vi "Read Measurements.vi"(8 "error in (no error)":errorcluster, 11 "PacificPowerSource in":refnum<class "PacificPowerSource.lvclass">) -> (0 "error out":errorcluster, 2 "BaseMeasurements":T1, 3 "PacificPowerSource out":refnum<class "PacificPowerSource.lvclass">)   [LabVIEW 2018, in "AcPwrPlugins.lvlib" / "PacificPowerSource.lvclass"]
uses:
  PacificPowerSource.lvclass
  TypeDefs/Measurements.ctl
  TypeDefs/MeasurementType.ctl
  PacificPowerSource.lvclass/PacificPowerSource.ctl
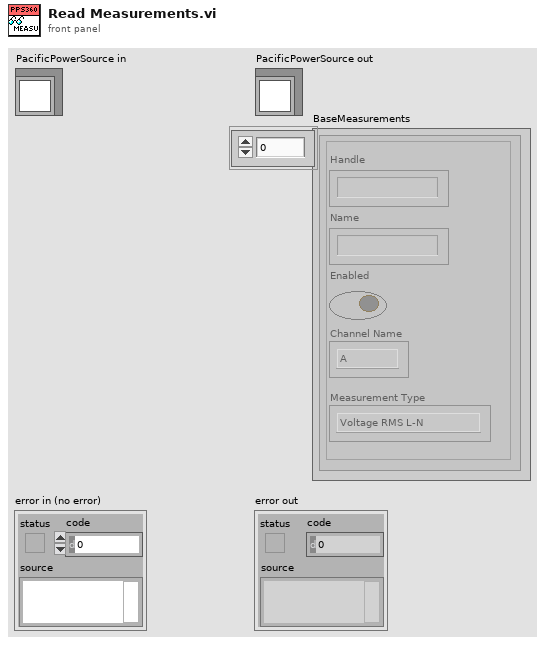
[diagram p1: front panel]
types:
  T1 = typedef "AcPwrPlugins.lvlib/PacificPowerSource.lvclass/Measurements.ctl" = cluster{"Handle":string, "Name":string, "Enabled ":bool, "Measurement Value":dbl, "Channel Name":enum16{"A", "B", "C"}, "Measurement Type ":T2}[]
  T2 = typedef "AcPwrPlugins.lvlib/PacificPowerSource.lvclass/MeasurementType.ctl" = enum16{"Voltage RMS L-N", "Voltage RMS L-L", "Frequency", "Current RMS", "Current Peak", "Crest Factor", "Power Factor", "Power VA", "Real Power"}
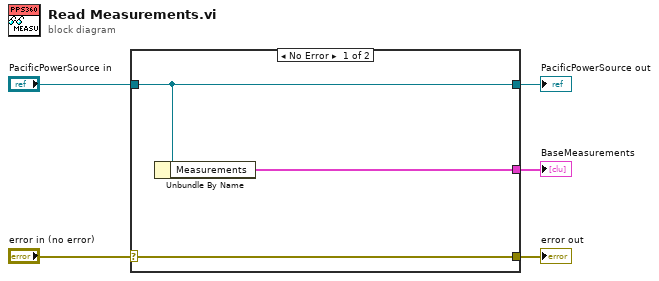
[diagram p0: block diagram]
diagram:
  n1 = case shown="No Error" "error in (no error)" {
    selector: "error in (no error)" -> [w8 w9]
    tunnel: [w8 w9] -> w4
    tunnel: [w7 w10] -> w2
    tunnel: "PacificPowerSource in" -> [w7 w10]
    tunnel: [w6 _] -> w1
    frame No Error {
      n2 = Unbundle By Name(w7) -> ("Measurements"=w6:T1)
    }
    frame Error {
    }
  }
  "error out" <- w4
  "PacificPowerSource out" <- w2
  "BaseMeasurements" <- w1
